vi "initregSG.vi"() -> (0 "Init Data Out":T1={"AOEnable"=FALSE, "AO0"=0, "SGUpdateRate"=40, "SGPhase"=0, "SGFreq"=100000, "SGAmp"=0, "SGSignalType"=0, "N"=0})   [LabVIEW 2013, in "IRIO.lvlib"]
uses:
  IRIO.lvlib
panel:
  # "For Initialization VI requirements and help, please read directions located on Block Diagram."
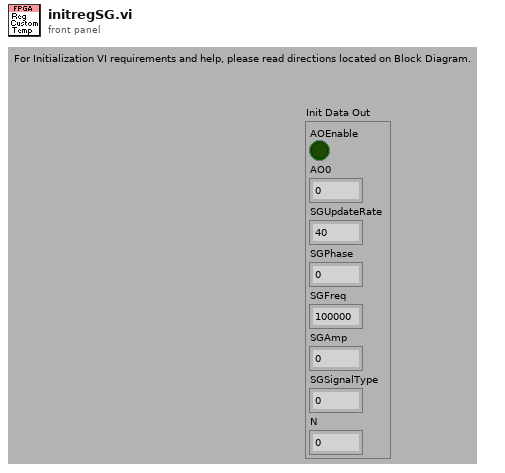
[diagram p1: front panel]
types:
  T1 = cluster{"AOEnable":bool, "AO0":i32, "SGUpdateRate":u32, "SGPhase":u32, "SGFreq":u32, "SGAmp":u16, "SGSignalType":u8, "N":u8}
  T2 = cluster{"AOEnable":bool, "AO0":i32, "SGUpdateRate":u32, "SGPhase":u32, "SGFreq":u32, "SGAmp":u16, "SGSignalType":u8, "N":i32}
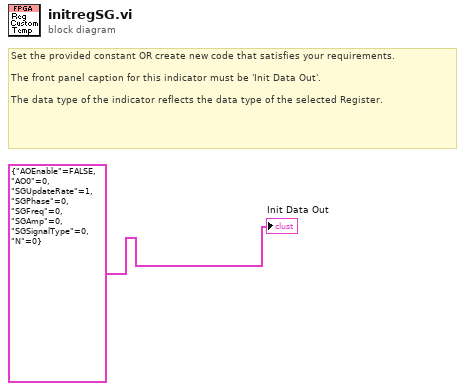
[diagram p0: block diagram]
diagram:
  # "Set the provided constant OR create new code that satisfies your requirements.\n\nThe front panel caption for this indicator must be 'Init Data Out'.\n\nThe data type of the indicator reflects the data type of the selected Register."
  "Init Data Out" <- T2 {"AOEnable"=FALSE, "AO0"=0, "SGUpdateRate"=1, "SGPhase"=0, "SGFreq"=0, "SGAmp"=0, "SGSignalType"=0, "N"=0} ("Cluster")
